vi "MAT.vi"(11 "Data in":T1) -> (3 "Data out":T1)   [LabVIEW 2022 SP3]
uses:
  controls/Data.ctl
panel:
  out "Volt nejis 2":dbl[](array[numeric])
  out "Curent nejis":dbl[](array[numeric])
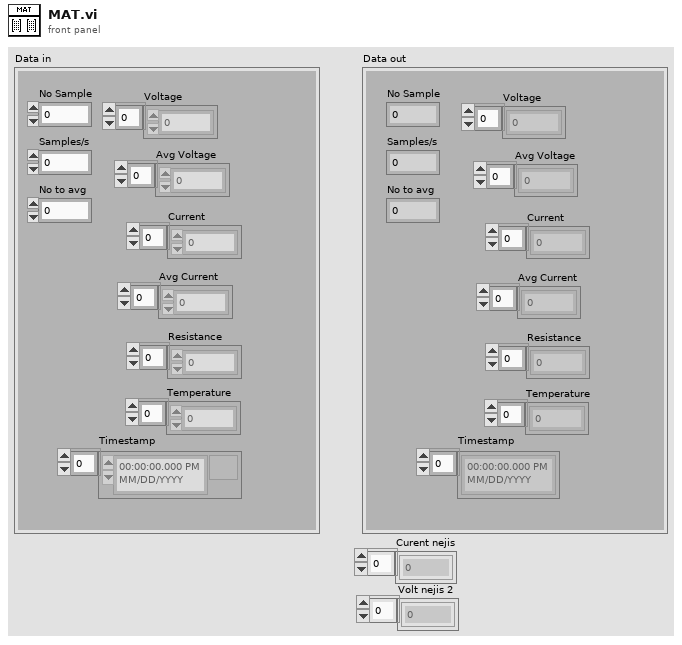
[diagram p1: front panel]
types:
  T1 = typedef "Data.ctl" = cluster{"No Sample":i32, "Samples/s":i32, "No to avg":i32, "Voltage":dbl[], "Current":dbl[], "Resistance":dbl[], "Temperature":dbl[], "Avg Voltage":dbl[], "Timestamp":timestamp[], "Avg Current":dbl[]}
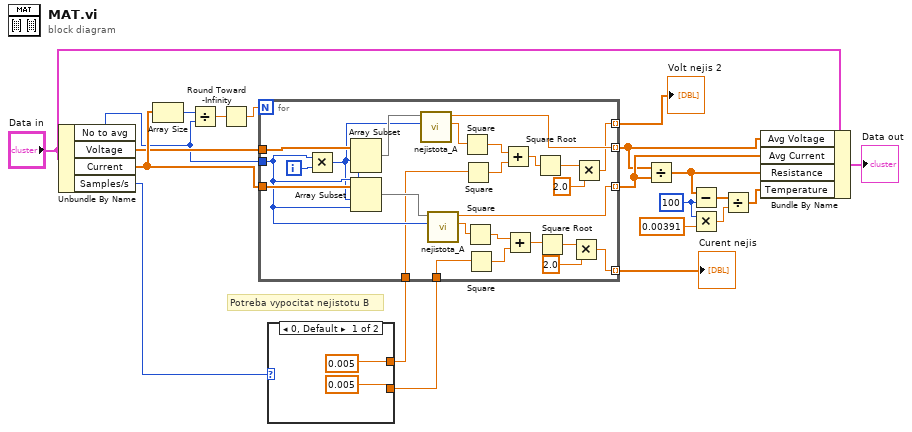
[diagram p0: block diagram]
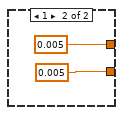
[diagram p2: hidden frame]
diagram:
  w14 = 100 ("mean")
  # "Potreba vypocitat nejistotu B"
  n1 = Unbundle By Name("Data in") -> ("No to avg"=w9:i32, "Voltage"=w20:dbl[], "Current"=w21:dbl[], "Samples/s"=w3:i32)
  n2 = Array Size(array=w21) -> (size(s)=w6:i32)
  n3 = Divide(x=w6, y=w9) -> (x/y=w7:dbl)
  n4 = Round Toward -Infinity(1:w7) -> (0:w8:dbl)
  n5 = case shown="0, Default" w3 {
    tunnel: [0.005 0.005] -> w2
    tunnel: [0.005 0.005] -> w1
    frame 0, Default {
    }
    frame 1 {
    }
  }
  n6 = for {
    N: w8 -> [_]
    tunnel: w20 -> [w50]
    tunnel: w9 -> [w45]
    tunnel: [w44] -> w16 mode=indexing
    tunnel: w21 -> [w48]
    tunnel: [w47] -> w17 mode=indexing
    tunnel: [w29] -> w5 mode=indexing
    tunnel: [w26] -> w4 mode=indexing
    tunnel: w2 -> [w33]
    tunnel: w1 -> [w32]
    i -> [w49]
    n7 = Multiply(x=w45, y=w49) -> (x*y=w42:i32)
    n8 = Array Subset(array=w50, index=w42, length=w45) -> (w43:dbl[])
    n9 = Array Subset(array=w48, index=w42, length=w45) -> (w46:dbl[])
    n10 = call "nejistota_A.vi"("No to avg"=w42, "Array"=w43) -> ("nejistota_A"=w40:dbl, "mean"=w44:dbl)  [unwired: 8 in]
    n11 = call "nejistota_A.vi"("No to avg"=w45, "Array"=w46) -> ("nejistota_A"=w41:dbl, "mean"=w47:dbl)  [unwired: 8 in]
    n12 = Square(x=w40) -> (x^2=w37:dbl)
    n13 = Square(x=w32) -> (x^2=w36:dbl)
    n14 = Square(x=w41) -> (x^2=w39:dbl)
    n15 = Square(x=w33) -> (x^2=w38:dbl)
    n16 = Add(x=w37, y=w36) -> (x+y=w35:dbl)
    n17 = Add(x=w39, y=w38) -> (x+y=w34:dbl)
    n18 = Square Root(x=w35) -> (sqrt(x)=w27:dbl)
    n19 = Square Root(x=w34) -> (sqrt(x)=w31:dbl)
    n20 = Multiply(x=w31, y=2.0) -> (x*y=w29:dbl)
    n21 = Multiply(x=w27, y=2.0) -> (x*y=w26:dbl)
  }
  "Curent nejis" <- w5
  "Volt nejis 2" <- w4
  n22 = Divide(x=w16, y=w17) -> (x/y=w18:dbl[])
  n23 = Subtract(x=w18, y=w14) -> (x-y=w15:dbl[])
  n24 = Multiply(x=w14, y=0.00391) -> (x*y=w12:dbl)
  n25 = Divide(x=w15, y=w12) -> (x/y=w19:dbl[])
  n26 = Bundle By Name(cluster="Data in", "Avg Voltage"=w16, "Avg Current"=w17, "Resistance"=w18, "Temperature"=w19) -> (→"Data out":T1)
